vi "计算散斑矩阵列平均值.vi"(1 "光源散斑簇":T1) -> (0 "散斑二维数组列平均值":dbl[](array[numeric]))   [LabVIEW 2018]
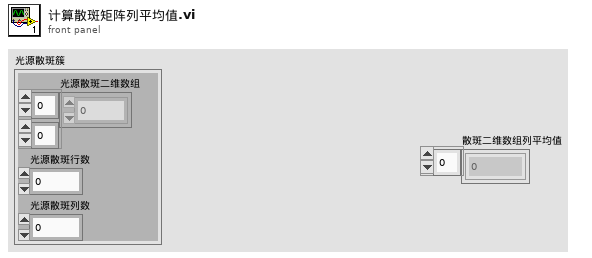
[diagram p1: front panel]
types:
  T1 = cluster{"光源散斑二维数组":dbl[][], "光源散斑行数":i32, "光源散斑列数":i32}
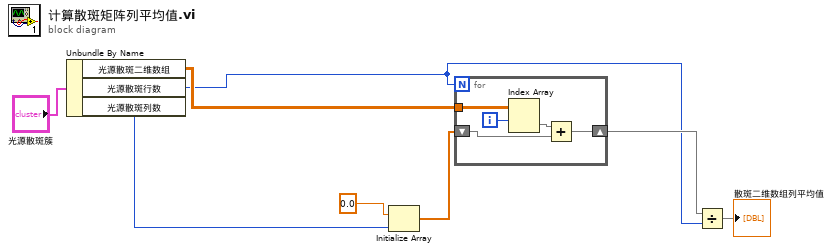
[diagram p0: block diagram]
diagram:
  n1 = Unbundle By Name("光源散斑簇") -> ("光源散斑二维数组"=w3:dbl[][], "光源散斑行数"=w2:i32, "光源散斑列数"=w1:i32)
  n2 = Initialize Array(0.0, w1) -> (w6:dbl[])
  n3 = for {
    N: w2 -> [_]
    shift-right: [w9] -> w8
    shift-left: w6 -> [w10]
    tunnel: w3 -> [w13]
    i -> [w12]
    n4 = Index Array(array=w13, index (row)=w12) -> (element=w11:dbl[])  [unwired: 1 in]
    n5 = Add(x=w11, y=w10) -> (x+y=w9:dbl[])
  }
  n6 = Divide(x=w8, y=w2) -> (x/y=→"散斑二维数组列平均值":dbl[])
